vi "initSound.vi"(0 "Error Message":string="Problemas al Inicializar el Sonido", 1 "Sound Parameters":T4) -> (2 "Sound Device OUT":T3 {"task ID" format="%.0x"}, 3 "# samples":u32, 4 "Inizializo?":bool, 5 "task ID":T1 format="%.0x")   [LabVIEW 2010]
uses:
  <vilib>/sound2/lvsound2.llb/Sound Data Format.ctl
  <vilib>/sound2/lvsound2.llb/Sound Output Task ID.ctl
  <vilib>/sound2/lvsound2.llb/Sampling Mode.ctl
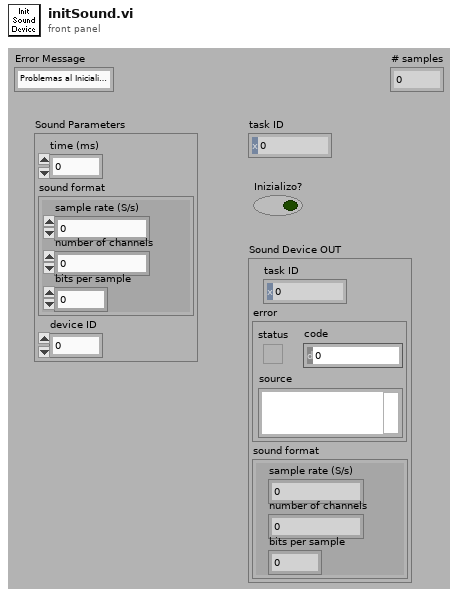
[diagram p1: front panel]
types:
  T1 = typedef "Sound Output Task ID.ctl" = u32
  T2 = typedef "Sound Data Format.ctl" = cluster{"sample rate (S/s)":dbl, "number of channels":i32, "bits per sample":i32}
  T3 = cluster{"task ID":T1, "error":errorcluster, "sound format":T2}
  T4 = cluster{"time (ms)":dbl, "sound format":T2, "device ID":u32}
  T5 = typedef "Sampling Mode.ctl" = i32
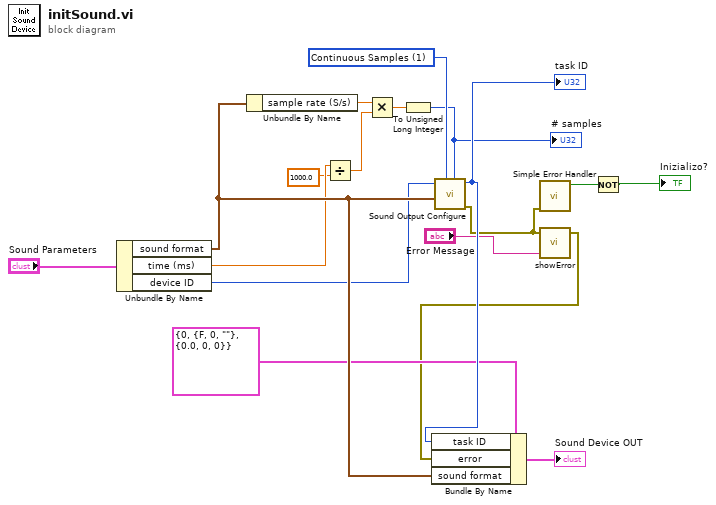
[diagram p0: block diagram]
diagram:
  w11 = T5 1 items=["Finite Samples", "Continuous Samples"] ("sample mode")
  n1 = Unbundle By Name("Sound Parameters") -> ("sound format"=w17:T2, "time (ms)"=w13:dbl, "device ID"=w12:u32)
  n2 = Unbundle By Name(w17) -> ("sample rate (S/s)"=w8:dbl)
  n3 = Divide(x=w13, y=sgl 1000.0) -> (x/y=w7:dbl)
  n4 = Multiply(x=w8, y=w7) -> (x*y=w10:dbl)
  n5 = To Unsigned Long Integer(number=w10) -> (unsigned 32bit integer=w6:u32)
  "# samples" <- w6
  n6 = call <vilib>:"Sound Output Configure.vi"("number of samples/ch"=w6, "sample mode"=w11, "sound format"=w17, "device ID"=w12) -> ("error out"=w1:errorcluster, "task ID"=w16:T1)  [unwired: 6 in]
  "task ID" <- w16
  n7 = call <vilib>:"Simple Error Handler.vi"("error in (no error)"=w1) -> ("error?"=w5:bool)  [unwired: 4 in, 4 out]
  n8 = call "showError.vi"("message"="Error Message", "Error IN"=w1) -> ("Error OUT"=w2:errorcluster)  [unwired: 3 in]
  n9 = Bundle By Name(cluster=T3 {"task ID"=0, "error"={"status"=FALSE, "code"=0, "source"=""}, "sound format"={"sample rate (S/s)"=0.0, "number of channels"=0, "bits per sample"=0}} ("Sound Device IN"), "task ID"=w16, "error"=w2, "sound format"=w17) -> (→"Sound Device OUT":T3)
  n10 = Not(x=w5) -> (.not. x?=→"Inizializo?":bool)
